vi "Dependency Change.vi"(5 "object ref in":T1, 7 "Column Change":i32, 8 "error in (no error)":errorcluster, 9 "new value":string, 10 "old value":string, 11 "Listbox TBDT in":refnum<class "Listbox TBDT.lvclass">) -> (0 "error out":errorcluster, 3 "Listbox TBDT out":refnum<class "Listbox TBDT.lvclass">)   [LabVIEW 2013]
uses:
  Listbox TBDT.lvclass
  TagSelectModule/Source/module/configuration/tag select module configuration.lvclass
  <vilib>/NI/Tag Bus Data Framework/Configuration Editor/Classes/Engine Parent/Engine Parent Editor Node.lvclass
  <vilib>/NI/Module Execution Interface/Engine Configuration/engine configuration.lvclass
  <vilib>/NI/Configuration Framework/serializable configuration/NISE_CEF_serializable configuration.lvclass
  <vilib>/NI/Tag Bus Data Framework/Configuration Editor/Classes/Module editor node/module editor node.lvclass
  <vilib>/NI/Tag Bus/tag/tag descriptor.lvclass
  TagSelectModule/Source/editor node/object ref.ctl
  TagSelectModule/Source/editor node/tag select module editor node.lvclass
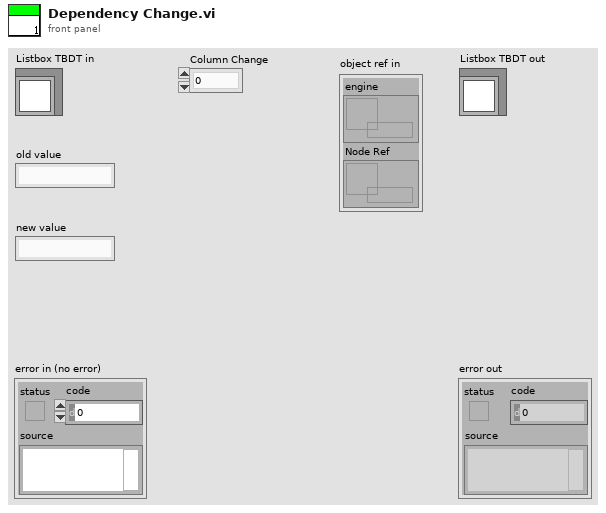
[diagram p1: front panel]
types:
  T1 = typedef "tag select module editor node.lvclass/object ref.ctl" = cluster{"engine":refnum<data-value>, "Node Ref":refnum<data-value>}
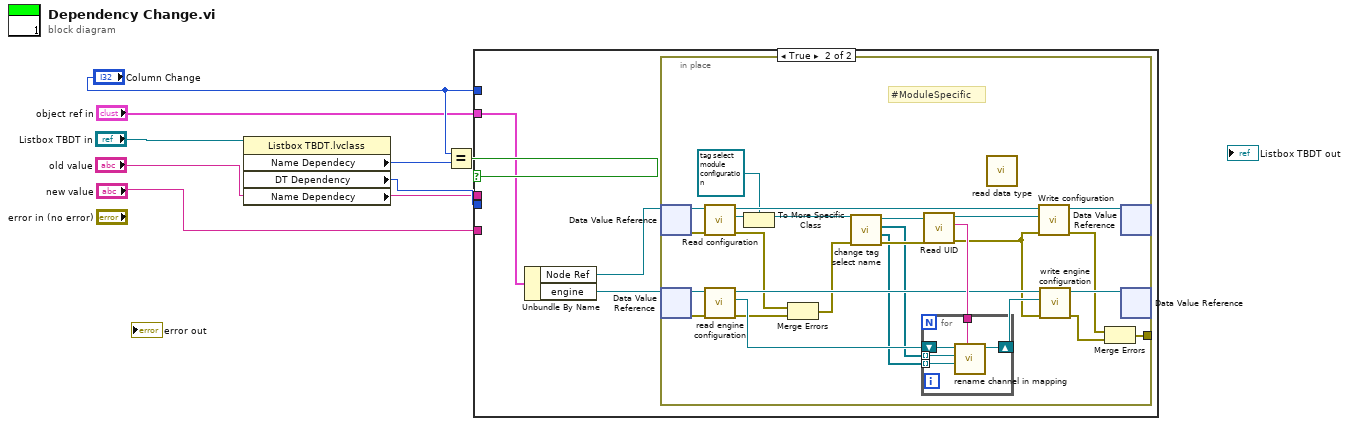
[diagram p0: block diagram]
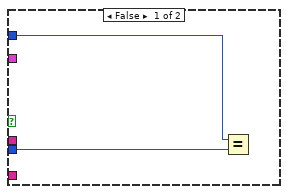
[diagram p2: hidden frame]
diagram:
  n1 = property class="Listbox TBDT.lvclass" props=["Name Dependecy", "DT Dependency", "Name Dependecy"](reference="Listbox TBDT in") -> ("Name Dependecy"=w7:i32, "DT Dependency"=w5:i32)  [unwired: 1 in, 3 out]
  n2 = Equal?(x="Column Change", y=w7) -> (x = y?=w6:bool)
  n3 = case shown="True" w6 {
    tunnel: w5 -> [w10 _]
    tunnel: "Column Change" -> [w9 _]
    tunnel: "object ref in" -> [_ w11]
    tunnel: "old value" -> [_ _]
    tunnel: "new value" -> [_ _]
    frame False {
      n4 = Equal?(x=w9, y=w10) -> ()  [unwired: 1 out]
    }
    frame True {
      n5 = Unbundle By Name(w11) -> ("Node Ref"=w12:refnum<data-value>, "engine"=w13:refnum<data-value>)
      n6 = in-place {
        in-place-border: [w26] -> _
        # "#ModuleSpecific"
        n7 = in-place-dvr #1(w12) -> (w20:refnum<class "module editor node.lvclass">, w25:errorcluster)
        n8 = in-place-dvr #2(w13) -> (w38:refnum<class "Engine Parent Editor Node.lvclass">, w39:errorcluster)
        n9 = call-dynamic "Read configuration.vi"("error in"=w25, "NISE_CEF_serializable node in"=w20) -> ("error out"=w24:errorcluster, "configuration"=w21:refnum<class "NISE_CEF_serializable configuration.lvclass">, "NISE_CEF_serializable node out"=w30:refnum<class "module editor node.lvclass">)  [unwired: 7 in]
        n10 = call <vilib>:"read engine configuration.vi"("error in"=w39, "Engine Parent Editor Node in"=w38) -> ("error out"=w33:errorcluster, "engine configuration"=w34:refnum<class "engine configuration.lvclass">, "Engine Parent Editor Node out"=w31:refnum<class "Engine Parent Editor Node.lvclass">)  [unwired: 7 in]
        n11 = To More Specific Class(target class=refnum<class "tag select module configuration.lvclass"> refnum ("tag select  module configuration in"), reference=w21) -> (specific class reference=w19:refnum<class "tag select module configuration.lvclass">)  [unwired: 1 in, 1 out]
        n12 = Merge Errors(w24, w33) -> (w18:errorcluster)
        n13 = call "change tag select name.vi"("error in"=w18, "tag select module configuration in"=w19) -> ("error out"=w17:errorcluster, "new channels"=w14:refnum<class "TBM channel.lvclass">[], "old channels"=w15:refnum<class "TBM channel.lvclass">[], "tag select module configuration out"=w16:refnum<class "tag select module configuration.lvclass">)  [unwired: 6 in]
        n14 = call <vilib>:"Read UID.vi"("error in"=w17, "configuration in"=w16) -> ("error out"=w23:errorcluster, "instance id"=w35:string, "configuration out"=w29:refnum<class "tag select module configuration.lvclass">)  [unwired: 7 in]
        n15 = for {
          shift-right: [w43] -> w32
          shift-left: w34 -> [w44]
          tunnel: w35 -> [w42]
          tunnel: w15 -> [w41] mode=indexing
          tunnel: w14 -> [w40] mode=indexing
          n16 = call <vilib>:"rename channel in mapping.vi"("owner ID"=w42, "new channel"=w40, "old channel"=w41, "engine configuration in"=w44) -> ("engine configuration out"=w43:refnum<class "engine configuration.lvclass">)  [unwired: 6 in, 1 out]
        }
        n17 = call <vilib>:"read data type.vi"() -> ()  [unwired: 9 in, 3 out]
        n18 = call-dynamic "Write configuration.vi"("error in"=w23, "configuration"=w29, "NISE_CEF_serializable node in"=w30) -> ("error out"=w27:errorcluster, "NISE_CEF_serializable node out"=w36:refnum<class "module editor node.lvclass">)  [unwired: 7 in]
        n19 = call <vilib>:"write engine configuration.vi"("error in"=w23, "engine configuration"=w32, "Engine Parent Editor Node in"=w31) -> ("error out"=w28:errorcluster, "Engine Parent Editor Node out"=w37:refnum<class "Engine Parent Editor Node.lvclass">)  [unwired: 7 in]
        n20 = Merge Errors(w27, w28) -> (w26:errorcluster)
        n21 = in-place-dvr #1(w36) -> ()  [unwired: 2 out]
        n22 = in-place-dvr #2(w37) -> ()  [unwired: 2 out]
      }
    }
  }
